vi "wordle.vi"   [LabVIEW 2017]
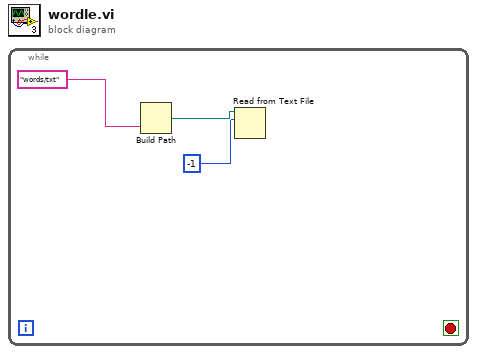
[diagram p0: block diagram]
diagram:
  n1 = while {
    stop <- _ stop-if-true
    n2 = Build Path(name or relative path="words/txt") -> (appended path=w2:path)  [unwired: 1 in]
    n3 = Read from Text File(file (use dialog)=w2, count=-1) -> ()  [unwired: 2 in, 4 out]
  }
